vi "get_voltage_and_current_set_low_limit.vi"(8 "error in":errorcluster, 11 "VISA resource name":refnum<visa-resource-name>="COM1") -> (0 "error out":errorcluster, 3 "Response":string)   [LabVIEW 2020]
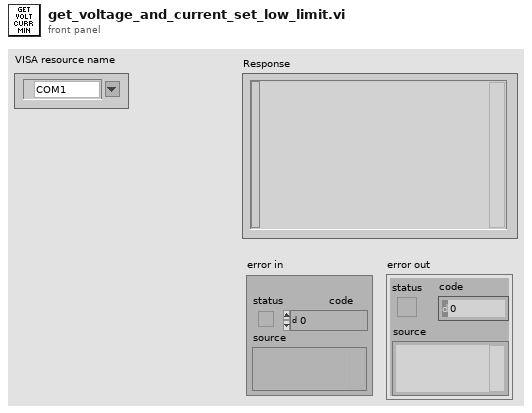
[diagram p1: front panel]
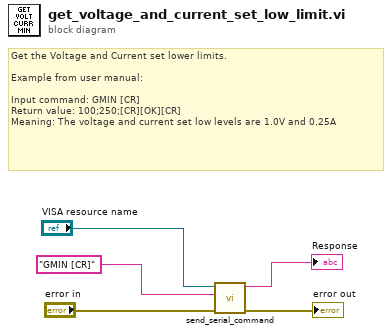
[diagram p0: block diagram]
diagram:
  # "Get the Voltage and Current set lower limits.\n\nExample from user manual:\n\nInput command: GMIN [CR]\nReturn value: 100;250;[CR][OK][CR]\nMeaning: The voltage and current set low levels are 1.0V and 0.25A"
  n1 = call "send_serial_command.vi"("error in (no error)"="error in", "Command"="GMIN [CR]", "VISA resource name"="VISA resource name") -> ("error out"=→"error out":errorcluster, "Response"=→"Response":string)  [unwired: 7 in]
